vi "centre of rotation 2.vi"(0 "Head rotation (Fick)":dbl[][](array[numeric]) format="%.2f", 1 "reference":i32, 7 "Analysis":enum16{"Instantaneous COR", "Average COR"}(ring), 11 "POSITION 3D":dbl[][](array[numeric]) format="%.2f") -> (4 "Coefficients":dbl[][](array[numeric]) format="%.2f", 15 "mse":dbl format="%.2f")   [LabVIEW 2016]
uses:
  <vilib>/Analysis/baseanly.llb/Real A x B.vi
  <vilib>/Analysis/_algsub.llb/Real PseudoInverse Matrix.vi
  <vilib>/Analysis/baseanly.llb/A x Vector.vi
  <vilib>/Analysis/baseanly.llb/Real Inverse Matrix.vi
  comm/fick-matrix/fick-matrix.lvlib
  <vilib>/Analysis/NI_AALBase.lvlib
  <vilib>/Analysis/NI_AALPro.lvlib
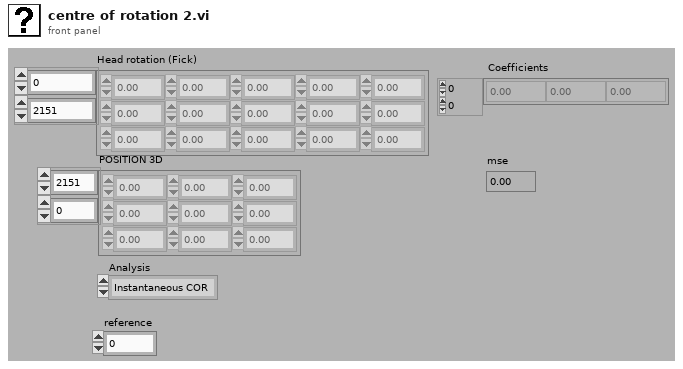
[diagram p1: front panel]
types:
  T1 = enum32{"SVD", "Givens", "Givens2", "Householder", "LU Decomposition", "Cholesky"}
  T2 = typedef "NI_Matrix.lvlib/RealMatrix.ctl" = dbl[][]
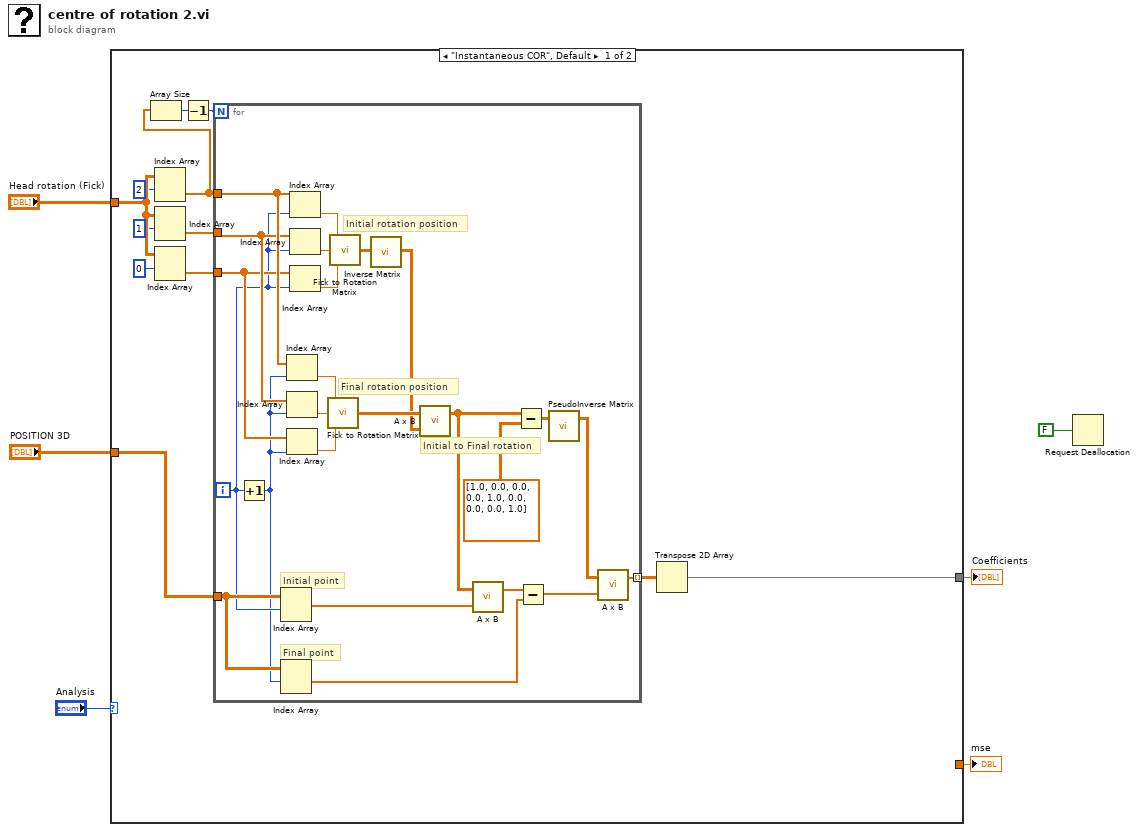
[diagram p0: block diagram]
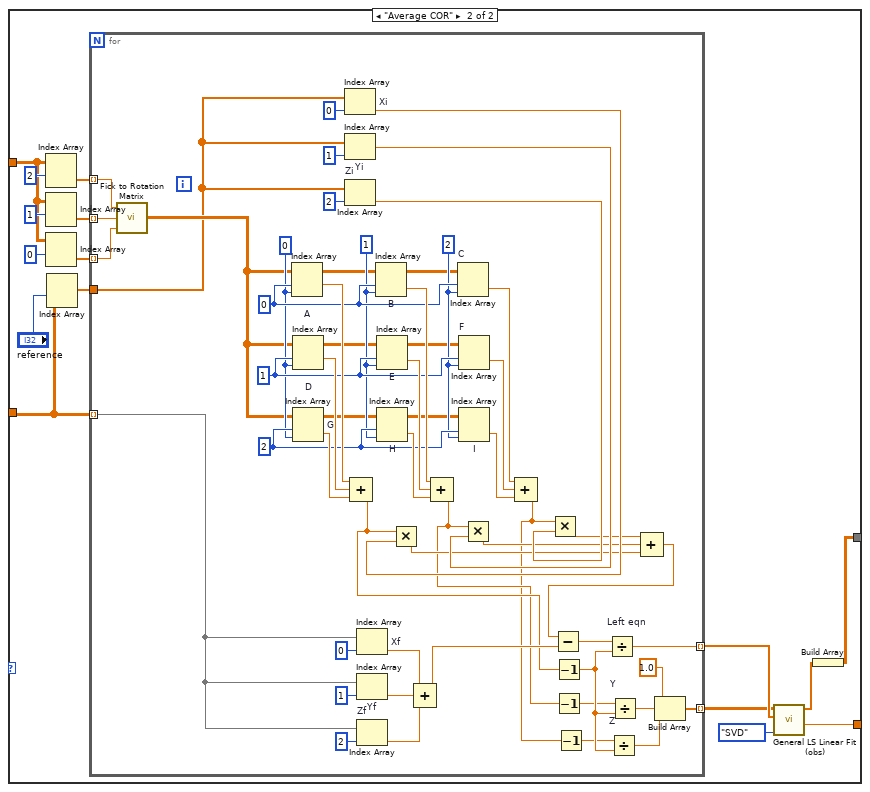
[diagram p2: hidden frame]
diagram:
  n1 = case shown="\"Instantaneous COR\", Default" "Analysis" {
    tunnel: "Head rotation (Fick)" -> [w19 w53]
    tunnel: "POSITION 3D" -> [w11 w49]
    tunnel: [0.0 ("mse") w52] -> w6
    tunnel: [w8 w50] -> w5
    frame "Instantaneous COR", Default {
      n2 = Index Array(array=w19, index (row)=2) -> (element=w12:dbl[])  [unwired: 1 in]
      n3 = Array Size(array=w12) -> (size(s)=w13:i32)
      n4 = Index Array(array=w19, index (row)=1) -> (element=w15:dbl[])  [unwired: 1 in]
      n5 = Index Array(array=w19, index (row)=0) -> (element=w14:dbl[])  [unwired: 1 in]
      n6 = Decrement(x=w13) -> (x-1=w10:i32)
      n7 = for {
        N: w10 -> [_]
        tunnel: w12 -> [w37]
        tunnel: w15 -> [w36]
        tunnel: w14 -> [w35]
        tunnel: w11 -> [w34]
        tunnel: [w25] -> w9 mode=indexing
        i -> [w33]
        # "Final rotation position"
        # "Initial rotation position"
        # "Final point"
        # "Initial point"
        # "Initial to Final rotation"
        n8 = Increment(x=w33) -> (x+1=w32:i32)
        n9 = Index Array(array=w34, index (row)=w33) -> (element=w31:dbl[])  [unwired: 1 in]
        n10 = Index Array(array=w34, index (row)=w32) -> (element=w29:dbl[])  [unwired: 1 in]
        n11 = Index Array(array=w37, index=w32) -> (element=w42:dbl)
        n12 = Index Array(array=w36, index=w32) -> (element=w43:dbl)
        n13 = Index Array(array=w35, index=w32) -> (element=w41:dbl)
        n14 = Index Array(array=w37, index=w33) -> (element=w39:dbl)
        n15 = Index Array(array=w36, index=w33) -> (element=w40:dbl)
        n16 = Index Array(array=w35, index=w33) -> (element=w38:dbl)
        n17 = call "Fick to Rotation Matrix.vi"("T"=w41, "V"=w43, "H"=w42) -> ("Rotation Matrix"=w24:dbl[][])
        n18 = call "Fick to Rotation Matrix.vi"("T"=w38, "V"=w40, "H"=w39) -> ("Rotation Matrix"=w23:dbl[][])
        n19 = call-poly <vilib>:"Inverse Matrix.vi"("Input Matrix"=w23) -> ("Inverse Matrix"=w22:T2)  [unwired: 1 in, 1 out]
        n20 = call-poly <vilib>:"A x B.vi"("B"=w22, "A"=w24) -> ("A x B"=w27:T2)  [unwired: 1 out]
        n21 = call-poly <vilib>:"A x B.vi"("Vector"=w31, "A"=w27) -> ("A x Vector"=w30:dbl[])  [unwired: 1 out]
        n22 = Subtract(x=w27, y=dbl[][] [[1.0, 0.0, 0.0], [0.0, 1.0, 0.0], [0.0, 0.0, 1.0]]) -> (x-y=w21:T2)
        n23 = Subtract(x=w30, y=w29) -> (x-y=w26:dbl[])
        n24 = call-poly <vilib>:"PseudoInverse Matrix.vi"("Input Matrix"=w21) -> ("PseudoInverse Matrix"=w20:T2)  [unwired: 1 in, 1 out]
        n25 = call-poly <vilib>:"A x B.vi"("Vector"=w26, "A"=w20) -> ("A x Vector"=w25:dbl[])  [unwired: 1 out]
      }
      n26 = Transpose 2D Array(2D array=w9) -> (transposed array=w8:dbl[][])
    }
    frame "Average COR" {
      n27 = Index Array(array=w53, index (row)=2) -> (element=w56:dbl[])  [unwired: 1 in]
      n28 = Index Array(array=w53, index (row)=1) -> (element=w55:dbl[])  [unwired: 1 in]
      n29 = Index Array(array=w53, index (row)=0) -> (element=w54:dbl[])  [unwired: 1 in]
      n30 = Index Array(array=w49, index (row)="reference") -> (element=w47:dbl[])  [unwired: 1 in]
      n31 = for {
        tunnel: w56 -> [w109] mode=indexing
        tunnel: w55 -> [w108] mode=indexing
        tunnel: w54 -> [w107] mode=indexing
        tunnel: [w79] -> w46 mode=indexing
        tunnel: [w75] -> w45 mode=indexing
        tunnel: w49 -> [w62] mode=indexing
        tunnel: w47 -> [w60]
        w69 = 2 ("disabled index (col)")
        w70 = 1 ("disabled index (col)")
        w74 = 2 ("index (row)")
        w73 = 1 ("index (row)")
        w71 = 0 ("disabled index (col)")
        w72 = 0 ("index (row)")
        n32 = call "Fick to Rotation Matrix.vi"("T"=w107, "V"=w108, "H"=w109) -> ("Rotation Matrix"=w61:dbl[][])
        n33 = Index Array "A"(array=w61, index (row)=w72, index (col)=w71) -> (element=w106:dbl)
        n34 = Index Array "D"(array=w61, index (row)=w73, index (col)=w71) -> (element=w105:dbl)
        n35 = Index Array "G"(array=w61, index (row)=w74, index (col)=w71) -> (element=w104:dbl)
        n36 = Index Array "Xi"(array=w60, index=0) -> (element=w94:dbl)
        n37 = Index Array "Yi"(array=w60, index=1) -> (element=w93:dbl)
        n38 = Index Array "Zi"(array=w60, index=2) -> (element=w92:dbl)
        n39 = Compound Arithmetic op=ADD(w106, w105, w104) -> (w86:dbl)
        n40 = Index Array "Xf"(array=w62, index=0) -> (element=w97:dbl)
        n41 = Index Array "Yf"(array=w62, index=1) -> (element=w96:dbl)
        n42 = Index Array "Zf"(array=w62, index=2) -> (element=w95:dbl)
        n43 = Index Array "B"(array=w61, index (row)=w72, index (col)=w70) -> (element=w103:dbl)
        n44 = Index Array "E"(array=w61, index (row)=w73, index (col)=w70) -> (element=w102:dbl)
        n45 = Index Array "H"(array=w61, index (row)=w74, index (col)=w70) -> (element=w101:dbl)
        n46 = Multiply(x=w86, y=w94) -> (x*y=w89:dbl)
        n47 = Compound Arithmetic op=ADD(w97, w96, w95) -> (w87:dbl)
        n48 = Compound Arithmetic op=ADD(w103, w102, w101) -> (w83:dbl)
        n49 = Index Array "C"(array=w61, index (row)=w72, index (col)=w69) -> (element=w100:dbl)
        n50 = Index Array "F"(array=w61, index (row)=w73, index (col)=w69) -> (element=w99:dbl)
        n51 = Index Array "I"(array=w61, index (row)=w74, index (col)=w69) -> (element=w98:dbl)
        n52 = Multiply(x=w83, y=w93) -> (x*y=w90:dbl)
        n53 = Compound Arithmetic op=ADD(w100, w99, w98) -> (w81:dbl)
        n54 = Multiply(x=w81, y=w92) -> (x*y=w91:dbl)
        n55 = Decrement(x=w86) -> (x-1=w84:dbl)
        n56 = Decrement(x=w83) -> (x-1=w82:dbl)
        n57 = Decrement(x=w81) -> (x-1=w80:dbl)
        n58 = Divide "Z"(x=w80, y=w84) -> (x/y=w76:dbl)
        n59 = Divide "Y"(x=w82, y=w84) -> (x/y=w77:dbl)
        n60 = Compound Arithmetic op=ADD(w91, w90, w89) -> (w88:dbl)
        n61 = Subtract(x=w88, y=w87) -> (x-y=w85:dbl)
        n62 = Divide "Left eqn"(x=w85, y=w84) -> (x/y=w79:dbl)
        n63 = Build Array(1.0 ("index (row)"), w77, w76) -> (w75:dbl[])
      }
      n64 = call <vilib>:"General LS Linear Fit (obs).vi"("H"=w45, "Y"=w46, "algorithm"=T1."SVD") -> ("Coefficients"=w51:dbl[], "mse"=w52:dbl)  [unwired: 2 in, 3 out]
      n65 = Build Array(w51) -> (w50:dbl[][])
    }
  }
  "mse" <- w6
  "Coefficients" <- w5
  n66 = Request Deallocation(FALSE ("flag")) -> ()
